vi "Get Wheel Information.vi"   [LabVIEW 2017, in "NI_Robotics_Wheel.lvclass"]
doc: "Returns information, such as <B>wheel radius</B> and <B>gear ratio</B>, for the wheel you specify. You must manually select the polymorphic instance to use."
uses:
  <vilib>/robotics/Steering/Wheel/NI_Robotics_Wheel.lvclass
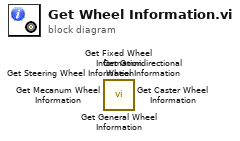
[diagram p0: block diagram]
diagram:
  n1 = call <vilib>:"Get General Wheel Information.vi"() -> ()  [unwired: 7 in, 5 out]
  n2 = call <vilib>:"Get Omnidirectional Wheel Information.vi"() -> ()  [unwired: 7 in, 5 out]
  n3 = call <vilib>:"Get Mecanum Wheel Information.vi"() -> ()  [unwired: 6 in, 6 out]
  n4 = call <vilib>:"Get Caster Wheel Information.vi"() -> ()  [unwired: 5 in, 7 out]
  n5 = call <vilib>:"Get Steering Wheel Information.vi"() -> ()  [unwired: 5 in, 7 out]
  n6 = call <vilib>:"Get Fixed Wheel Information.vi"() -> ()  [unwired: 7 in, 5 out]
